vi "Que Data To Process.vi"(7 "queue in":refnum<queue>, 8 "error in (no error)":errorcluster, 9 "PIFOC Pos":dbl, 10 "timestamp (nm)":i64, 11 "pDataBuffer in":u16[](array[numeric])) -> (0 "error out":errorcluster, 5 "queue out":refnum<queue>)   [LabVIEW 2020]
uses:
  _Controls/Logging Queue Cluster.ctl
  _Controls/Tweezertron Ctrl Refs.ctl
  _Controls/Confocal Controls.ctl
  _Controls/iFlex.ctl
  _Controls/PIFOC Position.ctl
  _Controls/Manlight Controls.ctl
  _Controls/Exp Params.ctl
  _Controls/Image Thresholds.ctl
  _Controls/Spots.ctl
  _Controls/Spot Params.ctl
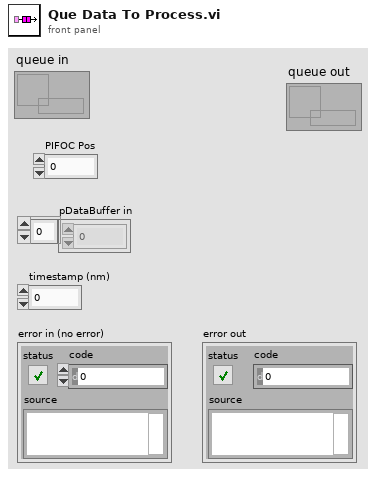
[diagram p1: front panel]
types:
  T1 = typedef "Logging Queue Cluster.ctl" = cluster{"message":string, "Data for Logging":cluster{"pDataBuffer":u16[], "timestamp (ns)":u64, "PI pos (um)":dbl}, "Tweezertron Ctrl Refs":T2}
  T2 = typedef "Tweezertron Ctrl Refs.ctl" = cluster{"LSM Settings":refnum<vi>, "iFlex Control":refnum<vi>, "PIFOC Settings":refnum<vi>, "PinSelector":refnum<vi>, "Manlight Controls":refnum<vi>, "Exp Params":refnum<vi>, "Image Thresholds":refnum<vi>, "RevFrame":refnum<vi>, "Spots":refnum<vi>}
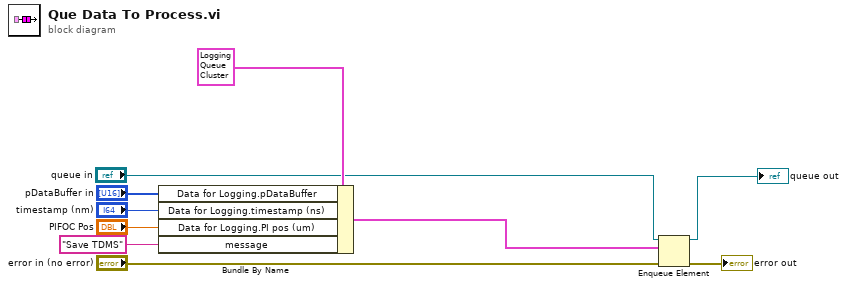
[diagram p0: block diagram]
diagram:
  n1 = Bundle By Name(cluster=T1 {"message"="", "Data for Logging"={"pDataBuffer"=[], "timestamp (ns)"=0, "PI pos (um)"=0.0}, "Tweezertron Ctrl Refs"={"LSM Settings"=refnum, "iFlex Control"=refnum, "PIFOC Settings"=refnum, "PinSelector"=refnum, "Manlight Controls"=refnum, "Exp Params"=refnum, "Image Thresholds"=refnum, "RevFrame"=refnum, "Spots"=refnum}} ("Logging Queue Cluster"), "Data for Logging.pDataBuffer"="pDataBuffer in", "Data for Logging.timestamp (ns)"="timestamp (nm)", "Data for Logging.PI pos (um)"="PIFOC Pos", "message"="Save TDMS" ("notification")) -> (w7:T1)
  n2 = Enqueue Element(queue="queue in", element=w7, error in (no error)="error in (no error)") -> (queue out=→"queue out":refnum<queue>, error out=→"error out":errorcluster)  [unwired: 1 in, 1 out]
